vi "sensor value data type.vi"(8 "error in (no error)":errorcluster, 10 "data_type_out":u32(ring)=98 items=["UHD_SENSOR_VALUE_BOOLEAN"=98, "UHD_SENSOR_VALUE_INTEGER"=105, "UHD_SENSOR_VALUE_REALNUM"=114, "UHD_SENSOR_VALUE_STRING"=115], 11 "h":u64) -> (0 "error out":errorcluster, 2 "data_type_out out":u32(ring)=98 items=["UHD_SENSOR_VALUE_BOOLEAN"=98, "UHD_SENSOR_VALUE_INTEGER"=105, "UHD_SENSOR_VALUE_REALNUM"=114, "UHD_SENSOR_VALUE_STRING"=115], 3 "function return":u32(ring))   [LabVIEW 2023, in "uhd.lvlib"]
doc: "UHD_API uhd_error uhd_sensor_value_data_type(\n uhd_sensor_value_handle h, uhd_sensor_value_data_type_t* data_type_out);"
uses:
  <userlib>/uhd/uhd.lvlib
  <userlib>/uhd/uhd.dll
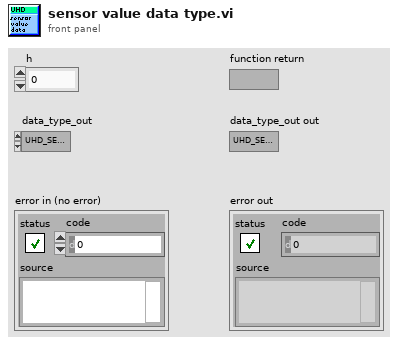
[diagram p1: front panel]
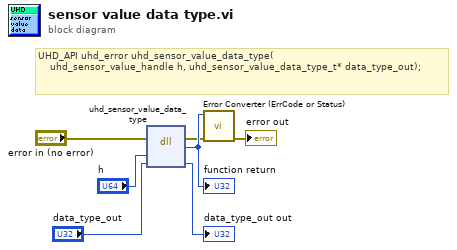
[diagram p0: block diagram]
diagram:
  # "UHD_API uhd_error uhd_sensor_value_data_type(\n    uhd_sensor_value_handle h, uhd_sensor_value_data_type_t* data_type_out);"
  n1 = dll-call lib="C:/Program Files/National Instruments/LabVIEW 2023/user.lib/uhd/uhd.*" fn="uhd_sensor_value_data_type"(error in="error in (no error)", "h"="h", "data_type_out"="data_type_out") -> (error out=w2:errorcluster, w7:u32, "data_type_out"=→"data_type_out out":u32)  [unwired: 3 in, 1 out]
  "function return" <- w7
  n2 = call <userlib>:"Error Converter (ErrCode or Status).vi"("error in (no error)"=w2, "error code"=w7) -> ("error out"=→"error out":errorcluster)  [unwired: 9 in]
